vi "pl1000SetInterval.vi"(0 "pl1000 handle":i16, 5 "usForBlock":u32, 7 "idealNoOfSamples":u32, 9 "channels":i16[](array[numeric]), 11 "error in (no error)":errorcluster) -> (4 "pl1000 handle out":i16, 15 "error out":errorcluster)   [LabVIEW 2016, in "pl1000.lvlib"]
doc: "This function sets the sampling rate of the unit. The fastest possible sampling interval is 1 microsecond, when the number of samples\nis 8192 divided by the number of channels active and the capture mode is BM_SINGLE. Under all other conditions, the fastest possible sampling interval is 10 microseconds per channel. The fastest possible data collection in the streaming settings is 100 kS/s (10 µs per sample), shared across all channels.\n\nus_for_block: target total time in which to collect\nideal_no_of_samples, in microseconds\n\nideal_no_of_samples: the total number of samples that you want\nto collect across all channels. This number is used only for timing\ncalculations\n\nchannels: an array of numbers identifying the channels from which\nyou wish to capture data"
uses:
  pl1000.lvlib
  pl1000.dll
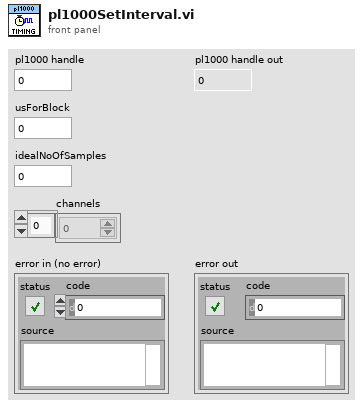
[diagram p1: front panel]
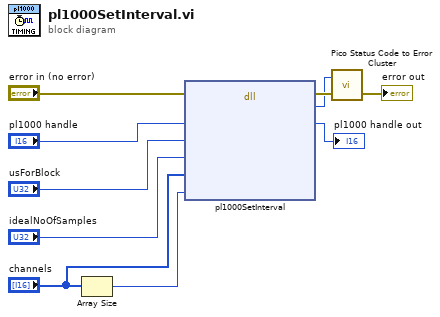
[diagram p0: block diagram]
diagram:
  n1 = Array Size(array="channels") -> (size(s)=w4:i32)
  n2 = dll-call lib="pl1000.dll" fn="pl1000SetInterval"(error in="error in (no error)", "handle"="pl1000 handle", "usForBlock"="usForBlock", "idealNoOfSamples"="idealNoOfSamples", "channels"="channels", "noOfChannels"=w4) -> (error out=w8:errorcluster, "status"=w7:u32, "handle"=→"pl1000 handle out":i16)  [unwired: 6 in, 1 out]
  n3 = call "Pico Status Code to Error Cluster.vi"("error in"=w8, "PICO_STATUS"=w7) -> ("error out"=→"error out":errorcluster)  [unwired: 1 in]
